vi "GetImage.vi"(0 "XRef":T15, 1 "State In":T3={"Worker Library Path"=path "", "Block Label"="", "Types"=[], "Selections"=[], "Icon"={"image type"=0, "image depth"=0, "image"=[], "mask"=[], "colors"=[], "Rectangle"={"left"=0, "top"=0, "right"=0, "bottom"=0}}, "Errors"={"Terminals"=[], "Generate"={"status"=FALSE, "code"=0, "source"=""}, "General"={"status"=FALSE, "code"=0, "source"=""}}, "Calculated Sizes"={"Block Width"=0, "Block Height"=0, "Half Width"=0, "Icon Top"=0, "Icon Bottom"=0, "Label Width"=0, "Half Label"=0, "Label Top"=0, "Text Width"=0, "Half Text"=0, "Text Height"=0, "Label Height"=0, "Expanded Width"=0, "Label Bottom"=0, "Expanded Top"=0, "Expanded Bottom"=0, "Expanded Height"=0, "Min Height"=0, "Max Height"=0}, "Special Terminal Indices"={"Action"=-1, "Init"=-1, "Tag"=-1, "State in"=-1, "State out"=-1, "Error"=-1, "Control"=-1, "Config"=-1}, "Terminals"=[], "Temp VI Name"="", "Description"="", "Smol Mode"=FALSE}) -> (14 "Image":T2, 15 "Fatal Error Out":T1)   [LabVIEW 2022 SP3, in "Flex Block.xnode"]
uses:
  Flex Block.xnode
  <vilib>/XNodeSupport/XNodeXNodeRef.ctl
  State.ctl
  FlexBlocks Support/Type Descriptor.ctl
  FlexBlocks Support/Terminal Direction.ctl
  FlexBlocks Support/Value Mode.ctl
  FlexBlocks Support/Special Terminal.ctl
  <vilib>/picture/picture.llb/imagedata.ctl
  FlexBlocks Support/XNode Errors.ctl
  FlexBlocks Support/Calculated Sizes.ctl
  FlexBlocks Support/Special Terminal Indices.ctl
  FlexBlocks Support/Terminal Status.ctl
  FlexBlocks Support/Terminal State.ctl
  FlexBlocks Support/Terminal Draw Style.ctl
  <vilib>/XNodeSupport/XNodeImage.ctl
  <vilib>/XNodeSupport/XNodeErrorCluster.ctl
  e085c9c5-5b4a-4080-8de0-22573a6995b1.vi
  FlexBlocks Support/_Add Ability Log.vi
  FlexBlocks Support/FlexBlocks Support.lvlib
  <vilib>/XNodeSupport/NI_XNodeSupport.lvlib
panel:
  out "new picture":picture
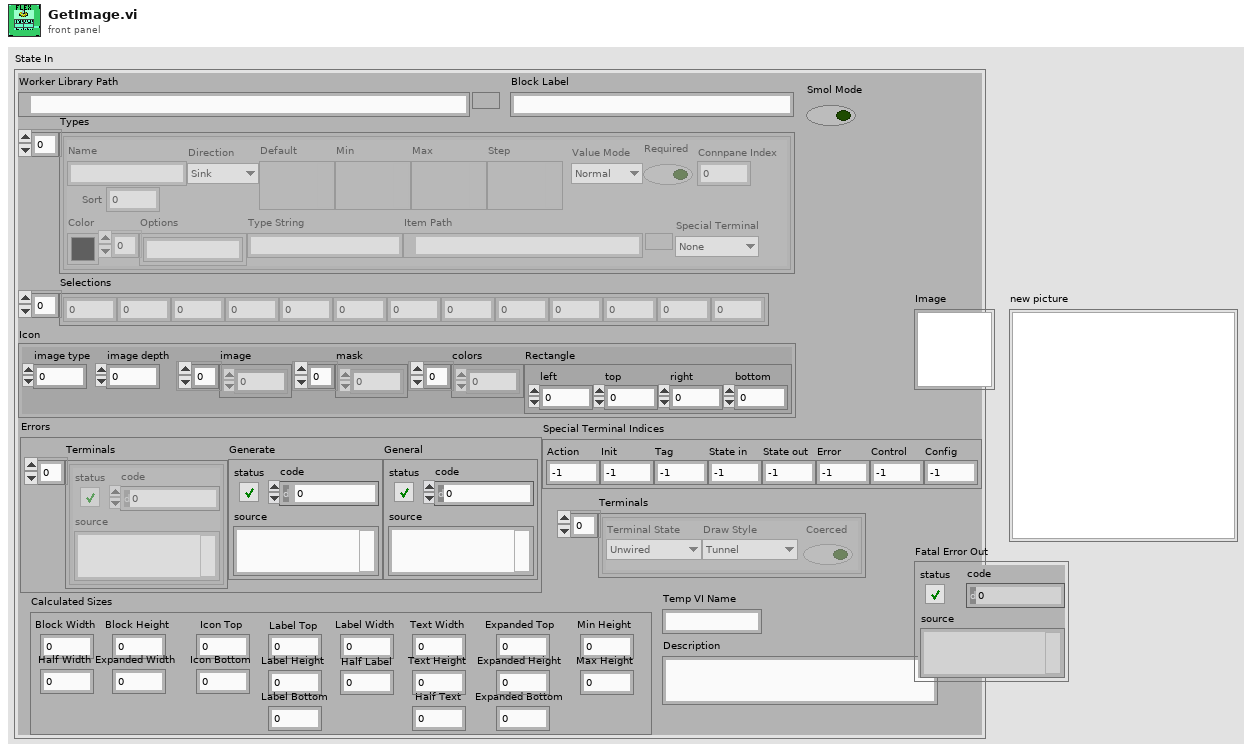
[diagram p1: front panel]
types:
  T1 = typedef "NI_XNodeSupport.lvlib/XNodeErrorCluster.ctl" = errorcluster
  T2 = typedef "NI_XNodeSupport.lvlib/XNodeImage.ctl" = picture
  T3 = typedef "Flex Block.xnode/State.ctl" = cluster{"Worker Library Path":path, "Block Label":string, "Types":T4[], "Selections":i32[], "Icon":T8, "Errors":T9, "Calculated Sizes":T10, "Special Terminal Indices":T11, "Terminals":T12[], "Temp VI Name":string, "Description":string, "Smol Mode":bool}
  T4 = typedef "FlexBlocks Support.lvlib/Type Descriptor.ctl" = cluster{"Name":string, "Direction":T5, "Default":variant, "Min":variant, "Max":variant, "Step":variant, "Value Mode":T6, "Color":u32, "Options":string[], "Type String":string, "Item Path":path, "Required":bool, "Connpane Index":i32, "Special Terminal":T7, "Sort":i32}
  T5 = typedef "FlexBlocks Support.lvlib/Terminal Direction.ctl" = enum16{"Sink", "Source"}
  T6 = typedef "FlexBlocks Support.lvlib/Value Mode.ctl" = enum16{"Normal", "Range", "Select"}
  T7 = typedef "FlexBlocks Support.lvlib/Special Terminal.ctl" = enum16{"None", "Action", "Init", "Tag", "State in", "State out", "Error", "Control", "Config"}
  T8 = typedef "imagedata.ctl" = cluster{"image type":i32, "image depth":i32, "image":u8[], "mask":u8[], "colors":u32[], "Rectangle":cluster{"left":i16, "top":i16, "right":i16, "bottom":i16}}
  T9 = typedef "FlexBlocks Support.lvlib/XNode Errors.ctl" = cluster{"Terminals":errorcluster[], "Generate":errorcluster, "General":errorcluster}
  T10 = typedef "FlexBlocks Support.lvlib/Calculated Sizes.ctl" = cluster{"Block Width":i32, "Block Height":i32, "Half Width":i32, "Icon Top":i32, "Icon Bottom":i32, "Label Width":i32, "Half Label":i32, "Label Top":i32, "Text Width":i32, "Half Text":i32, "Text Height":i32, "Label Height":i32, "Expanded Width":i32, "Label Bottom":i32, "Expanded Top":i32, "Expanded Bottom":i32, "Expanded Height":i32, "Min Height":i32, "Max Height":i32}
  T11 = typedef "FlexBlocks Support.lvlib/Special Terminal Indices.ctl" = cluster{"Action":i32, "Init":i32, "Tag":i32, "State in":i32, "State out":i32, "Error":i32, "Control":i32, "Config":i32}
  T12 = typedef "FlexBlocks Support.lvlib/Terminal Status.ctl" = cluster{"Terminal State":T13, "Draw Style":T14, "Coerced":bool}
  T13 = typedef "FlexBlocks Support.lvlib/Terminal State.ctl" = enum16{"Unwired", "BadType", "BadRef", "Channel", "Value", "Control Ref"}
  T14 = typedef "FlexBlocks Support.lvlib/Terminal Draw Style.ctl" = enum16{"Tunnel", "BadType", "BadRef", "Channel", "Value", "Control Ref"}
  T15 = typedef "NI_XNodeSupport.lvlib/XNodeXNodeRef.ctl" = refnum<vi>
  T16 = cluster{"left":i16, "top":i16, "right":i16, "bottom":i16}
  T17 = typedef "FlexBlocks Support.lvlib/Size Constants.ctl" = cluster{"Icon Size":i32, "Name H Pad":i32, "Name V Pad":i32, "Max Label Width":i32, "Value Width":i32, "Frame Padding":i32, "Vertical Margin":i32, "Min Width":i32, "Min Height":i32, "Collapsed Spacing":i32, "Terminal Center Offset":i32}
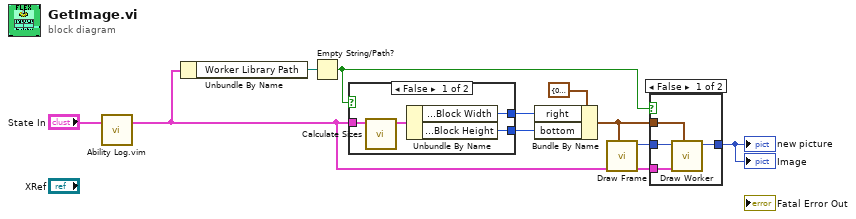
[diagram p0: block diagram]
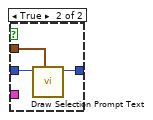
[diagram p2: hidden frame]
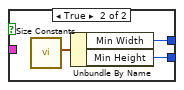
[diagram p3: hidden frame]
diagram:
  n1 = call "Ability Log.vim"("Wire in"="State In") -> ("Wire out"=w1:T3)  [unwired: 6 in]
  n2 = Unbundle By Name(w1) -> ("Worker Library Path"=w9:path)
  n3 = Empty String/Path?(string/path=w9) -> (empty?=w5:bool)
  n4 = case shown="False" w5 {
    tunnel: [w13 w16] -> w8
    tunnel: [w12 w15] -> w7
    tunnel: w1 -> [w11 _]
    frame False {
      n5 = call "Calculate Sizes.vi"("State In"=w11) -> ("State"=w14:T3)  [unwired: 10 in]
      n6 = Unbundle By Name(w14) -> ("Calculated Sizes.Block Width"=w13:i32, "Calculated Sizes.Block Height"=w12:i32)
    }
    frame True {
      n7 = call "Size Constants.vi"() -> ("Size Constants"=w17:T17)  [unwired: 11 in]
      n8 = Unbundle By Name(w17) -> ("Min Width"=w16:i32, "Min Height"=w15:i32)
    }
  }
  n9 = Bundle By Name(cluster=T16 {"left"=0, "top"=0, "right"=180, "bottom"=200} ("Bounds"), "right"=w8, "bottom"=w7) -> (w3:T16)
  n10 = call "Draw Frame.vi"("Bounds"=w3) -> ("Picture"=w6:picture)  [unwired: 10 in]
  n11 = case shown="False" w5 {
    tunnel: w6 -> [w21 w24]
    tunnel: [w19 w23] -> w4
    tunnel: w3 -> [w20 w22]
    tunnel: w1 -> [w18 _]
    frame False {
      n12 = call "Draw Worker.vi"("Bounds"=w20, "State"=w18, "Picture In"=w21) -> ("Picture"=w19:picture)  [unwired: 8 in]
    }
    frame True {
      n13 = call "Draw Selection Prompt Text.vi"("Bounds"=w22, "Picture In"=w24) -> ("Picture"=w23:picture)  [unwired: 9 in]
    }
  }
  "Image" <- w4
  "new picture" <- w4
